vi "Soft_Robot_Model.vi"() -> ()   [LabVIEW 2015]
uses:
  <vilib>/addons/Control Design/_Model Construction/Model Typedefs.llb/CD State Space Model (MIMO).ctl
  <vilib>/addons/Control Design/_Model Construction/Model Typedefs.llb/CD General Elements.ctl
  <vilib>/Platform/TimedLoop/XDataNode/timing_clust.ctl
  <vilib>/Platform/TimedLoop/XDataNode/nitl_modes.ctl
  <vilib>/Platform/TimedLoop/XDataNode/wakeup.ctl
  <vilib>/Analysis/7linalg.llb/Create Special Real Matrix.vi
  <vilib>/addons/Control Design/_Model Construction/Model Creation.llb/Model Creation SubVI/cd_Create State Space Model.vi
  <vilib>/addons/Control Design/_Stochastic Systems/Stochastic Systems.llb/CD Construct Noise Model (Numeric).vi
  <vilib>/addons/Control Design/_State Feedback Control/State Feedback Control.llb/State Feedback Control SubVis/cd_Discretized Linear Quadratic Regulator.vi
  <vilib>/Simulation/Estimation/Implementation/NILVSim Discrete Kalman Filter.llb/SIM Disc KF Pred and Corr with Pred Gain with Checking Direct LV.vi
  <vilib>/addons/Control Design/_State Feedback Control/State Feedback Control.llb/CD State Compensator.vi
  <vilib>/FPGAPlugInAG/myRIO-1900/niLvFpga_Open_myRIO-1900.vi
  <vilib>/rvi/interface/common/dynamic/niFpgaDynamicAddResources.vi
  <vilib>/Utility/error.llb/Error Cluster From Error Code.vi
  <vilib>/rvi/errors/niLvFpgaAdjustHostInterfaceError.vi
  <vilib>/FPGAPlugInAG/Dynamic/niLvFpga_Close_Dynamic.vi
  <vilib>/Platform/TimedLoop/XDataNode/XDataNode.xnode
  <vilib>/Simulation/Implementation/XNodeFramework/SimXNode/SimX.xnode
  <vilib>/rvi/interface/nirviOpenFPGA/nirviOpenFPGA.xnode
  FPGA Bitfiles/ACC20115_FPGATarget_CurrentControlle_Dt5vFgOzYtY.lvbitx
  Current Controller.vi
  <vilib>/rvi/interface/nirviReadWriteControl/nirviReadWriteControl.xnode
  <vilib>/rvi/interface/nirviCloseFPGA/nirviCloseFPGA.xnode
  <vilib>/addons/Control Design/_Model Construction/NI_LinSys_Model Creation.lvlib
  <vilib>/addons/Control Design/_State Feedback Control/NI_CD_State Feedback Control.lvlib
  <vilib>/addons/Control Design/_Stochastic Systems/NI_CD_Stochastic Systems.lvlib
  <vilib>/Analysis/NI_AALPro.lvlib
  <vilib>/Platform/TimedLoop/XDataNode/XDNodeRunTimeDep.lvlib
  NiFpgaLv.dll
  <vilib>/rvi/interface/Simulation/niFpgaSimulationCallBeginRW.vi
  <vilib>/addons/Control Design/_Model Construction/NI_LinSys_Model Typedefs.lvlib
panel:
  in  "LQR Output  matrix (R)  2":dbl[](array[numeric])
  in  "SP1: 2":dbl(slide)=40.87020302841148 min=0.0 max=0.0 scale=0.0..720.0
  in  "Tab Control":enum32{"Outputs", "Inputs"}(tab)
  out "Fusion Data":dbl(graph)
  out "KF estimate":dbl[](graph)
  in  "Stop":bool
  out "DAC Inlet Valve 2":i32(graph)
  in  "Current (mA)":i32
  out "Status?":bool
  out "State-Space Model":T1 {"Transport Delay" format="%.2f"; "D" format="%#.2g"; "C" format="%#.2g"; "B" format="%#.2g"; "A" format="%#.2g"; "properties"."Sampling Time" format="%#.6p"; "properties"."Output Delays" format="%.4f"; "properties"."Input Delays" format="%.4f"}
  out "Kalman Filter Gain M(k)":dbl[][](array[numeric])
  in  "LQR Matrix (Q)":dbl[](array[slide])=[1.133823501217849, 15.19911082952933] scale=0.001..1000.0
  in  "LQR Output  matrix (R)":dbl[](array[slide]) scale=0.0001..10.0
  in  "xhat(0|-1)":dbl[](array[numeric])=[1.0, 0.0]
  in  "Cov P(0|-1)":dbl[][](array[numeric])=[[1.0, 0.0], [0.0, 1.0]]
  out "xhat(k|k)":dbl[](array[numeric])
  out "xhat(k+1|k)":dbl[](array[numeric])
  in  "A":dbl[][](array[numeric]) format="%#.5g"
  in  "B":dbl[][](array[numeric]) format="%#.5g"
  in  "C":dbl[][](array[numeric]) format="%#.5g"
  in  "KF Q":dbl[][](array[numeric])=[[0.01, 0.0], [0.0, 0.001]]
  in  "KF R":dbl[][](array[numeric])=[[0.1]]
  in  "E{v}":dbl[](array[numeric]) format="%#.2g"
  in  "E{w}":dbl[](array[numeric]) format="%#.2g"
  in  "G":dbl[][](array[numeric]) format="%#.2g"
  out "error out":errorcluster
  in  "Desired CL Poles":cdb[](array[numeric]) format="%.3f"
  out "Actual CL Poles":cdb[](array[numeric]) format="%.3f"
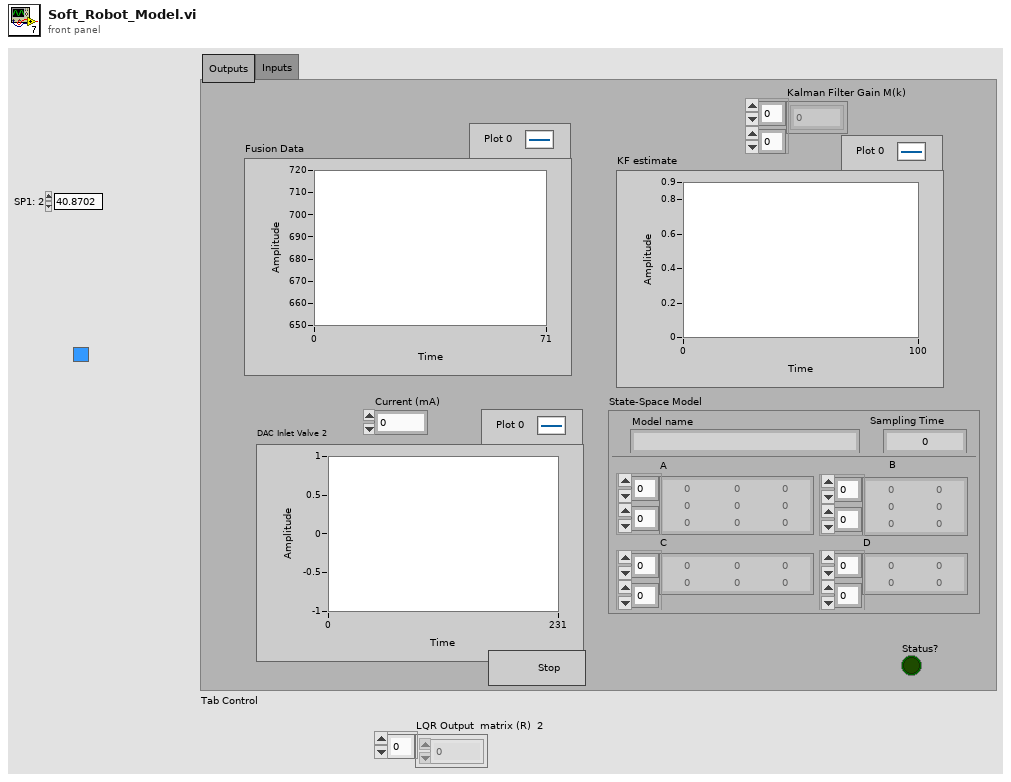
[diagram p1: front panel]
types:
  T1 = typedef "NI_LinSys_Model Typedefs.lvlib/CD State Space Model (MIMO).ctl" = cluster{"properties":T2, "A":dbl[][], "B":dbl[][], "C":dbl[][], "D":dbl[][], "StateNames":string[], "Transport Delay":dbl[][]}
  T2 = typedef "NI_LinSys_Model Typedefs.lvlib/CD General Elements.ctl" = cluster{"Model name":string, "Input names":string[], "Output names":string[], "Input Delays":dbl[], "Output Delays":dbl[], "Sampling Time":dbl, "Notes":string}
  T3 = typedef "XDNodeRunTimeDep.lvlib/timing_clust.ctl" = cluster{"Expected End [f-1]":u64, "Actual End [f-1]":u64, "Finished Late? [f-1]":bool, "Expected End [i-1]":u64, "Actual End [i-1]":u64, "Finished Late? [i-1]":bool, "Expected Start [i]":u64, "Actual Start [i]":u64, "Expected Start [f]":u64, "Actual Start [f]":u64, "Source Name":string, "Structure Name":string, "Period":i64, "Deadline":i64, "Offset":i64, "Start":i64, "Priority":i32, "Timeout":i32, "Mode":T4, "Wakeup Reason":T5, "Error":errorcluster, "Source Type":string, "Secondary Source Type":string, "Global End Time":u64, "Global Start Time":u64, "Frame Duration":u64, "Iteration Duration":u64, "Assigned CPU":i32, "I/O Scan Engine Mode":u32}
  T4 = typedef "XDNodeRunTimeDep.lvlib/nitl_modes.ctl" = enum32{"No Change", "Process missed periods, maintain original phase", "Discard missed periods, maintain original phase", "Process missed periods, ignore original phase", "Discard missed periods, ignore original phase"}
  T5 = typedef "XDNodeRunTimeDep.lvlib/wakeup.ctl" = enum32{"Normal", "Aborted", "Asynchronous wakeup", "Timing source error", "Timed loop error", "Timeout"}
  T6 = enum16{"state weighting", "output weighting, Dim Q = Ny", "output weighting, Dim Q = Nx"}
  T7 = enum32{"Identity", "Diagonal", "Toepliz", "Vandermonde", "Companion"}
  T8 = typedef "NI_Matrix.lvlib/RealMatrix.ctl" = dbl[][]
  T9 = typedef "NI_CD_Stochastic Systems.lvlib/cd_Stochastic State-Space Model.ctl" = cluster{"Sampling Time (s)":dbl, "G":dbl[][], "B":dbl[][], "A":dbl[][], "C":dbl[][], "D":dbl[][], "H":dbl[][]}
  T10 = typedef "NI_CD_Stochastic Systems.lvlib/cd_Second-Order Statistics Noise Model.ctl" = cluster{"Q":dbl[][], "E{w}":dbl[], "E{v}":dbl[], "R":dbl[][], "N":dbl[][]}
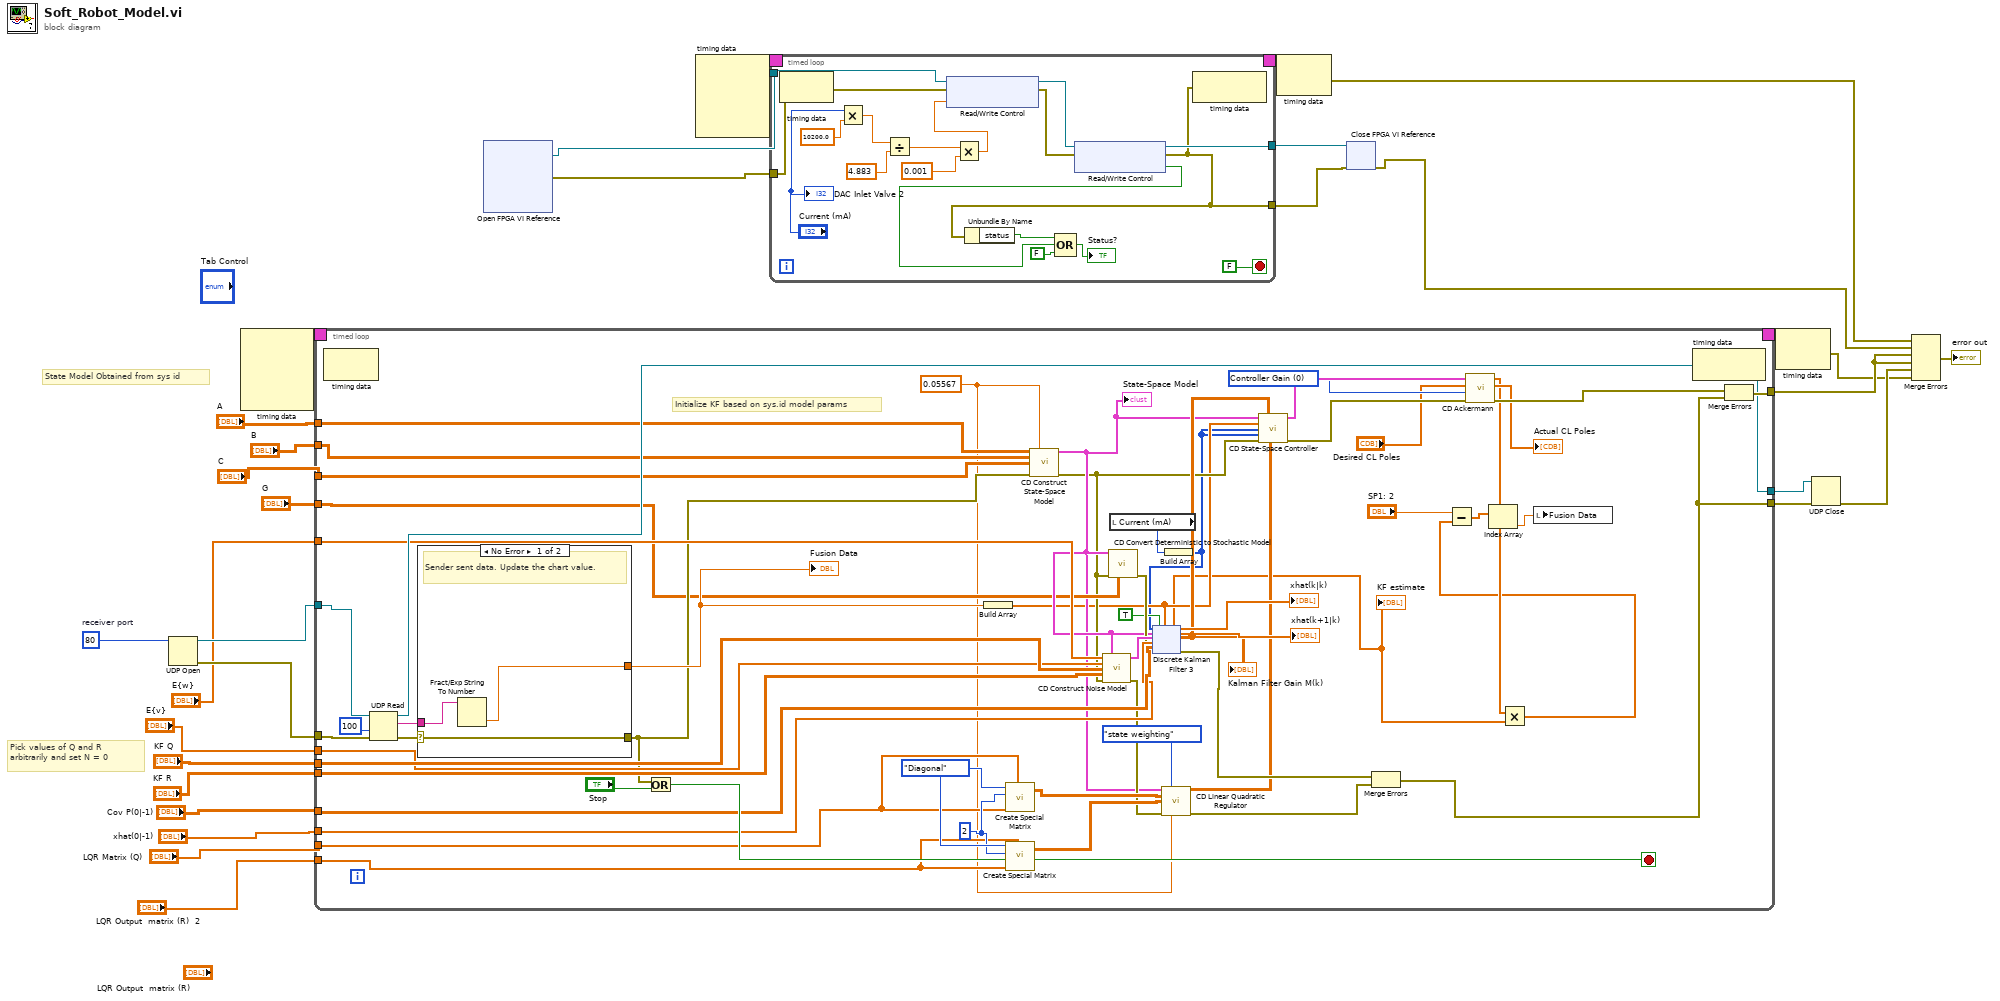
[diagram p0: block diagram]
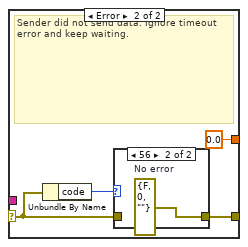
[diagram p2: hidden frame]
diagram:
  w29 = u16 80  # receiver port
  # "Pick values of Q and R\narbitrarily and set N = 0"
  # "State Model Obtained from sys id"
  n1 = UDP Open(11:w29) -> (port=w28:refnum<k16>, 0:w27:errorcluster)  [unwired: 4 in, 1 out]
  n2 = node-c288() -> (w13:T3)  [unwired: 4 in]
  n3 = timed-loop {
    tunnel: [w77] -> w24
    tunnel: w28 -> [w72]
    tunnel: w27 -> [w71]
    tunnel: [w68] -> w26
    tunnel: "A" -> [w67]
    tunnel: "B" -> [w66]
    tunnel: "C" -> [w65]
    tunnel: "KF Q" -> [w64]
    tunnel: "KF R" -> [w63]
    tunnel: "Cov P(0|-1)" -> [w62]
    tunnel: "xhat(0|-1)" -> [w61]
    tunnel: "E{v}" -> [w60]
    tunnel: "E{w}" -> [w59]
    tunnel: "LQR Matrix (Q)" -> [w52]
    tunnel: "LQR Output  matrix (R)  2" -> [w51]
    timing: w13 -> [_]
    timing-out: [_] -> w12
    tunnel: "G" -> [w54]
    tunnel: [w49] -> w4
    stop <- w69 stop-if-true
    w41 = u16 0 items=["Controller Gain", "Observer Gain (Predictive)", "Observer Gain (Current)"] ("Gain Type")
    w81 = 2
    w86 = T7."Diagonal" ("matrix type")
    w50 = 0.05567 ("Sampling Time (s)")
    # "Initialize KF based on sys.id model params"
    n4 = node-c288() -> ()  [unwired: 1 in, 1 out]
    n5 = UDP Read(connection ID=w72, timeout ms (25000)=100, 8:w71) -> (data out=w74:string, error out=w73:errorcluster, 3:w68:refnum<k16>)  [unwired: 3 out]
    n6 = case shown="No Error" w73 {
      selector: w73 -> [w93 w97]
      tunnel: w74 -> [w94 _]
      tunnel: [w93 w96] -> w58
      tunnel: [w92 0.0] -> w70
      frame No Error {
        # "Sender sent data. Update the chart value."
        n7 = Fract/Exp String To Number(string=w94) -> (number=w92:dbl)  [unwired: 3 in, 1 out]
      }
      frame Error {
        # "Sender did not send data. Ignore timeout error and keep waiting."
        n8 = Unbundle By Name(w97) -> ("code"=w98:i32)
        n9 = case shown="56" w98 {
          tunnel: w97 -> [w99 _]
          tunnel: [w99 w100] -> w96
          frame Default {
          }
          frame 56 {
            w100 = errorcluster {"status"=FALSE, "code"=0, "source"=""}  # No error
          }
        }
      }
    }
    "Fusion Data" <- w70
    n10 = Or(x=w58, y="Stop") -> (x .or. y?=w69:bool)
    n11 = Build Array ("Build Array 6")(w70) -> (w45:dbl[])
    n12 = call-poly <vilib>:"Create Special Matrix.vi"("matrix type"=w86, "matrix size"=w81, "Input Vector1"=w52, "Input Vector2"=w52) -> ("Special Matrix"=w84:T8)  [unwired: 1 in, 1 out]
    n13 = call-poly <vilib>:"Create Special Matrix.vi"("matrix type"=w86, "matrix size"=w81, "Input Vector1"=w51, "Input Vector2"=w51) -> ("Special Matrix"=w83:T8)  [unwired: 1 in, 1 out]
    n14 = call-poly <vilib>:"CD Construct State-Space Model.vi"("A"=w67, "Sampling Time (s)"=w50, "B"=w66, "C"=w65, "error in (no error)"=w58) -> ("State-Space Model"=w47:T1, "error out"=w46:errorcluster)  [unwired: 9 in]
    "State-Space Model" <- w47
    n15 = call <vilib>:"CD Convert Deterministic to Stochastic Model.vi"("Deterministic State-Space Model"=w47, "error in (no error)"=w46, "G"=w54) -> ("Stochastic State-Space Model"=w55:T9, "error out"=w56:errorcluster)  [unwired: 11 in]
    n16 = call-poly <vilib>:"CD Construct Noise Model.vi"("E{w}"=w59, "Stochastic State-Space Model"=w55, "E{v}"=w60, "Q"=w64, "R"=w63, "error in (no error)"=w46) -> ("Second-Order Statistics Noise Model out"=w79:T10, "error out"=w57:errorcluster)  [unwired: 8 in]
    n17 = local read "Current (mA)"() -> (w88:i32)
    n18 = call-poly <vilib>:"CD Linear Quadratic Regulator.vi"("Continuous State-Space Model"=w47, "Weighting Type"=T6."state weighting", "Q"=w84, "R"=w83, "error in (no error)"=w57, "Sampling Time (s)"=w50) -> ("Optimal Gain (K)"=w37:dbl[][], "error out"=w82:errorcluster)  [unwired: 6 in, 2 out]
    n19 = Build Array ("Build Array 5")(w88) -> (w44:i32[])
    n20 = xnode ("Discrete Kalman Filter 3")("input u(k)"=w44, "Stochastic State-Space Model"=w55, "Second-Order Statistics Noise Model"=w79, "Initial State Estimate xhat(0|-1)"=w61, "Initial Estimation Error Covariance P(0|-1)"=w62, "Initialize?"=TRUE, "Output y(k)"=w45, "error in (no error)"=w56) -> ("Estimated Output yhat(k)"=w35:dbl[], "Corrected State Estimate xhat(k|k)"=→"xhat(k|k)":dbl[], "Predicted State Estimate xhat(k+1|k)"=→"xhat(k+1|k)":dbl[], "Kalman Filter Gain M(k)"=w48:dbl[][], "error out"=w87:errorcluster)  [unwired: 3 out]
    "KF estimate" <- w35
    "Kalman Filter Gain M(k)" <- w48
    n21 = call-poly <vilib>:"CD State-Space Controller.vi"("State-Space Model"=w47, "Estimator Gain (L)"=w48, "Measured Outputs"=w45, "Known Inputs"=w44, "Manipulated Inputs"=w44, "error in (no error)"=w46, "Controller Gain (K)"=w37) -> ("Controller Model"=w43:T1, "error out"=w42:errorcluster)  [unwired: 7 in]
    n22 = Merge Errors(w87, w82) -> (w49:errorcluster)
    n23 = call <vilib>:"CD Ackermann.vi"("error in (no error)"=w42, "Gain Type"=w41, "Poles"="Desired CL Poles", "State-Space Model"=w43) -> ("error out"=w40:errorcluster, "Actual Poles"=→"Actual CL Poles":cdb[], "Gain"=w36:dbl[])  [unwired: 5 in]
    n24 = Multiply(x=w36, y=w35) -> (x*y=w34:dbl[])
    n25 = Subtract(x="SP1: 2", y=w34) -> (x-y=w33:dbl[])
    n26 = Index Array(array=w33) -> (element=w32:dbl)  [unwired: 1 in]
    n27 = local write "Fusion Data"(w32) -> ()
    n28 = node-c288() -> ()  [unwired: 1 in, 1 out]
    n29 = Merge Errors(w40, w49) -> (w77:errorcluster)
  }
  n30 = xnode "Open FPGA VI Reference"() -> ("FPGA VI Reference Out"=w10:refnum<k20>, "error out"=w9:errorcluster)  [unwired: 2 in]
  n31 = node-c288() -> (w8:T3)  [unwired: 4 in]
  n32 = timed-loop {
    tunnel: w10 -> [w133]
    tunnel: w9 -> [w118]
    tunnel: [w117] -> w30
    tunnel: [w126] -> w31
    timing: w8 -> [_]
    timing-out: [_] -> w7
    stop <- FALSE stop-if-true
    n33 = node-c288() -> ()  [unwired: 1 in, 1 out]
    n34 = Multiply(x="Current (mA)", y=10200.0) -> (x*y=w121:dbl)
    n35 = Divide(x=w121, y=4.883) -> (x/y=w124:dbl)
    n36 = Multiply(x=w124, y=0.001) -> (x*y=w120:dbl)
    n37 = xnode "Read/Write Control"("FPGA VI Reference In"=w133, "error in"=w118, "DAC Inlet Valve"=w120) -> ("FPGA VI Reference Out"=w132:refnum<k20>, "error out"=w131:errorcluster)
    n38 = xnode "Read/Write Control"("FPGA VI Reference In"=w132, "error in"=w131) -> ("FPGA VI Reference Out"=w126:refnum<k20>, "error out"=w117:errorcluster, "Inlet Overflow?"=w127:bool)
    n39 = Unbundle By Name(w117) -> ("status"=w129:bool)
    n40 = Compound Arithmetic op=OR(w129, w127, FALSE ("value")) -> (→"Status?":bool)
    n41 = node-c288(w117) -> ()  [unwired: 1 out]
    "DAC Inlet Valve 2" <- "Current (mA)"
  }
  n42 = node-c288(w7) -> (w5:errorcluster)
  n43 = xnode "Close FPGA VI Reference"("FPGA VI Reference In"=w31, "error in"=w30) -> ("error out"=w6:errorcluster)
  n44 = node-c288(w12) -> (w3:errorcluster)
  n45 = UDP Close(connection ID=w26, 8:w4) -> (error out=w25:errorcluster)  [unwired: 1 out]
  n46 = Merge Errors(w5, w6, w24, w24, w25, w3) -> (→"error out":errorcluster)
